vi "cv.to.local_volume.vi"(5 "volume":i32, 7 "volume type":T1=enum."One Shot" caption="Enum", 8 "error in (no error)":errorcluster, 11 "cv volume":T2) -> (0 "error out":errorcluster, 3 "local volume":T6={"id"=0, "name"="", "sortable_name"="", "aliases"=[], "description"="", "site_detail_url"="", "count_of_issues"=0, "start_year"=0, "publisher_id"=0, "issue_ids"=[], "date_last_updated"=timestamp(0 s since 1904-01-01), "volume"=0, "cv_id"="", "volume type"=enum."One Shot"})   [LabVIEW 2024, in "CV_RESTful_Lib.lvlib"]
uses:
  CV_RESTful_Lib.lvlib
  typedefs/local_volume--cluster.ctl
  CV_Shared_Library/volume.type--enum.ctl
  typedefs/cv_volume--cluster.ctl
  typedefs/cv_volume.results--cluster.ctl
  typedefs/cv_volume.issue--cluster.ctl
  typedefs/cv_volume.publisher--cluster.ctl
  <vilib>/Utility/error.llb/Trim Whitespace One-Sided.vi
  <userlib>/_OpenG.lib/string/string.llb/openg_string.lvlib
  CV_Shared_Library/CV_Shared_Library.lvlib
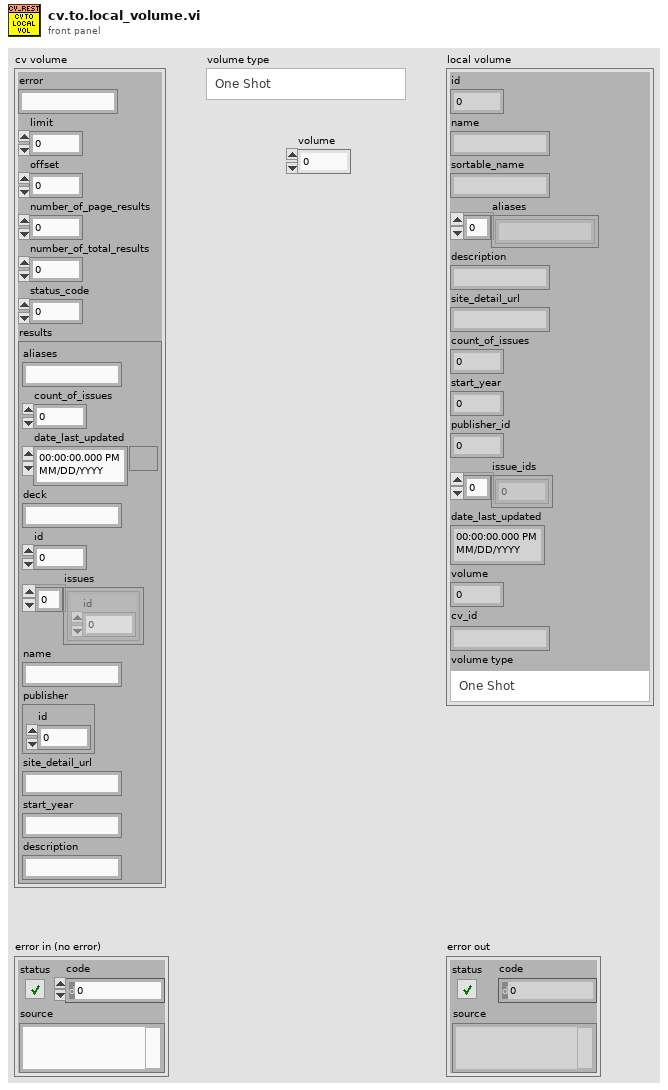
[diagram p1: front panel]
types:
  T1 = typedef "CV_Shared_Library.lvlib/volume.type--enum.ctl" = enum16{"Ongoing", "Limited Series", "Annual", "One Shot", "Reprint/Document", "Star Comics", "Epic Comics"}
  T2 = typedef "CV_RESTful_Lib.lvlib/cv_volume--cluster.ctl" = cluster{"error":string, "limit":i32, "offset":i32, "number_of_page_results":i32, "number_of_total_results":i32, "status_code":i32, "results":T3}
  T3 = typedef "CV_RESTful_Lib.lvlib/cv_volume.results--cluster.ctl" = cluster{"aliases":string, "count_of_issues":i32, "date_last_updated":timestamp, "deck":string, "id":i32, "issues":T4[], "name":string, "publisher":T5, "site_detail_url":string, "start_year":string, "description":string}
  T4 = typedef "CV_RESTful_Lib.lvlib/cv_volume.issue--cluster.ctl" = cluster{"id":i32}
  T5 = typedef "CV_RESTful_Lib.lvlib/cv_volume.publisher--cluster.ctl" = cluster{"id":i32}
  T6 = typedef "CV_RESTful_Lib.lvlib/local_volume--cluster.ctl" = cluster{"id":i32, "name":string, "sortable_name":string, "aliases":string[], "description":string, "site_detail_url":string, "count_of_issues":i32, "start_year":i32, "publisher_id":i32, "issue_ids":i32[], "date_last_updated":timestamp, "volume":i32, "cv_id":string, "volume type":T1}
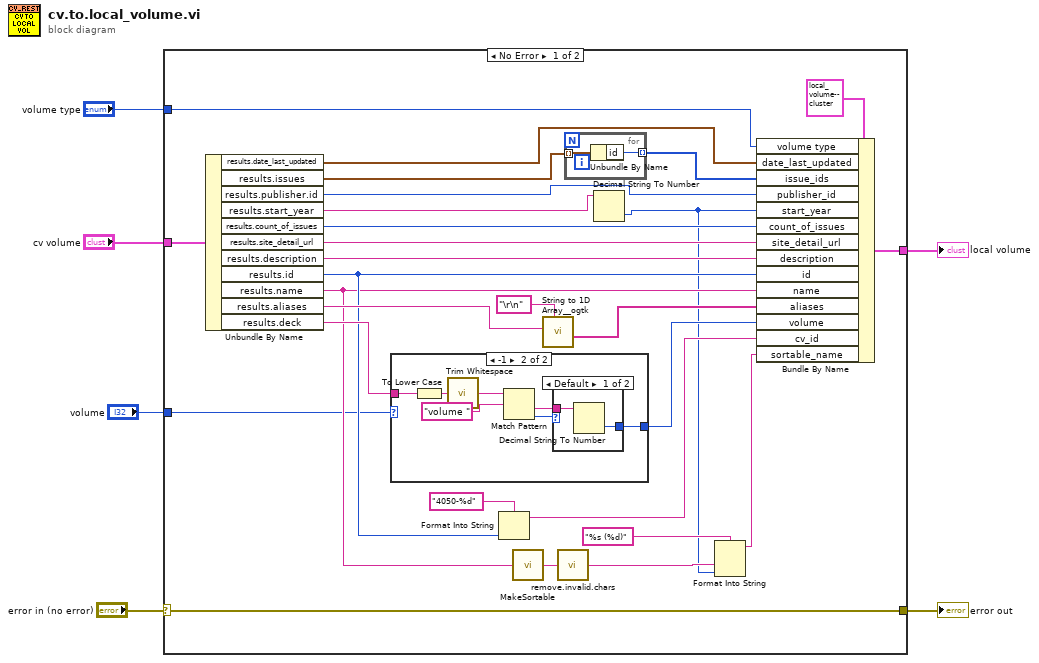
[diagram p0: block diagram]
diagram:
  n1 = case shown="No Error" "error in (no error)" {
    selector: "error in (no error)" -> [w7 w47]
    tunnel: "cv volume" -> [w33 _]
    tunnel: [w32 _] -> w5
    tunnel: "volume type" -> [w13 _]
    tunnel: "volume" -> [w8 _]
    tunnel: [w7 w47] -> w1
    frame No Error {
      n2 = Unbundle By Name(w33) -> ("results.date_last_updated"=w20:timestamp, "results.issues"=w22:T4[], "results.publisher.id"=w23:i32, "results.start_year"=w24:string, "results.count_of_issues"=w25:i32, "results.site_detail_url"=w26:string, "results.description"=w27:string, "results.id"=w16:i32, "results.name"=w14:string, "results.aliases"=w30:string, "results.deck"=w19:string)
      n3 = case shown="-1" w8 {
        selector: w8 -> [w35 _]
        tunnel: w19 -> [_ w42]
        tunnel: [w35 w36] -> w18
        frame Default {
        }
        frame -1 {
          n4 = To Lower Case(string=w42) -> (all lower case string=w41:string)
          n5 = call <vilib>:"Trim Whitespace.vi"("string"=w41) -> ("trimmed string"=w40:string)  [unwired: 1 in]
          n6 = Match Pattern(string=w40, regular expression="volume ") -> (after substring=w37:string, offset past match=w38:i32)  [unwired: 1 in, 2 out]
          n7 = case shown="Default" w38 {
            tunnel: w37 -> [w44 _]
            tunnel: [w43 _] -> w36
            frame Default {
              n8 = Decimal String To Number(string=w44) -> (number=w43:i32)  [unwired: 2 in, 1 out]
            }
            frame -1 {
            }
          }
        }
      }
      n9 = Format Into String(format string="4050-%d", w16) -> (resulting string=w15:string)  [unwired: 2 in, 1 out]
      n10 = call "MakeSortable.vi"("string in"=w14) -> ("string out"=w31:string)
      n11 = call <userlib>:"String to 1D Array__ogtk.vi"("delimiter (Tab)"="\r\n", "string"=w30) -> ("Array of Strings"=w28:string[])  [unwired: 9 in]
      n12 = call "remove.invalid.chars.vi"("string in"=w31) -> ("string out"=w11:string)
      n13 = for {
        tunnel: w22 -> [w46] mode=indexing
        tunnel: [w45] -> w21 mode=indexing
        n14 = Unbundle By Name(w46) -> ("id"=w45:i32)
      }
      n15 = Decimal String To Number(string=w24) -> (number=w10:i32)  [unwired: 2 in, 1 out]
      n16 = Format Into String(format string="%s (%d)", w11, w10) -> (resulting string=w9:string)  [unwired: 2 in, 1 out]
      n17 = Bundle By Name(cluster=T6 {"id"=0, "name"="", "sortable_name"="", "aliases"=[], "description"="", "site_detail_url"="", "count_of_issues"=0, "start_year"=0, "publisher_id"=0, "issue_ids"=[], "date_last_updated"=timestamp(0 s since 1904-01-01), "volume"=0, "cv_id"="", "volume type"=enum."One Shot"} ("volume"), "volume type"=w13, "date_last_updated"=w20, "issue_ids"=w21, "publisher_id"=w23, "start_year"=w10, "count_of_issues"=w25, "site_detail_url"=w26, "description"=w27, "id"=w16, "name"=w14, "aliases"=w28, "volume"=w18, "cv_id"=w15, "sortable_name"=w9) -> (w32:T6)
    }
    frame Error {
    }
  }
  "local volume" <- w5
  "error out" <- w1
